vi "Append Horizontal Line to Report.vi"(4 "noshade (F)":bool, 5 "width units":enum16{"Pixels", "Percentage"}(ring), 6 "size (default)":i32=-1, 7 "error in (no error)":errorcluster, 8 "width (0=default)":dbl format="%.2f", 9 "align (default)":T2, 10 "report in":T1) -> (0 "error out":errorcluster, 3 "report out":T1)   [LabVIEW 2015]
doc: "Creates a horizontal rule in an HTML report. You cannot use this VI with standard reports."
uses:
  <vilib>/Utility/NIReport.llb/HTML Report Text Alignment.ctl
  <vilib>/Utility/NIReport.llb/Generate Report Object Reference.ctl
  <vilib>/Utility/NIReport.llb/NI_report.lvclass
  <vilib>/Utility/NIReport.llb/NI_ReportGenerationCore.lvlib
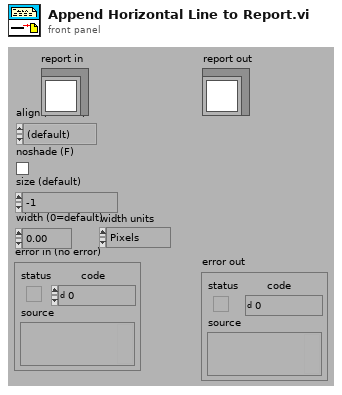
[diagram p1: front panel]
types:
  T1 = typedef "Generate Report Object Reference.ctl" = refnum<class "NI_report.lvclass">
  T2 = typedef "NI_ReportGenerationCore.lvlib/HTML Report Text Alignment.ctl" = enum16{"(default)", "LEFT", "CENTER", "RIGHT"}
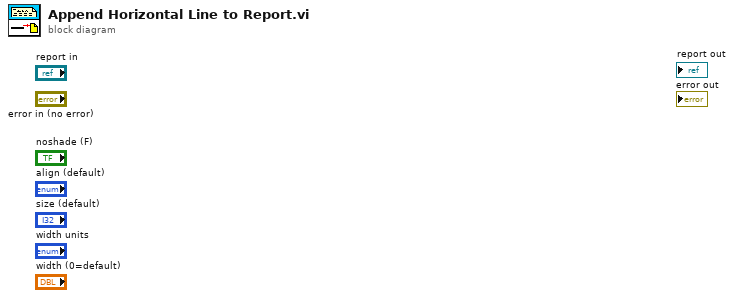
[diagram p0: block diagram]
diagram:
